vi "Delete Items.vi"(6 "indent":i32, 8 "error in (no error)":errorcluster, 9 "Copy? (F)":bool, 10 "Indices to remove":i32[](array[numeric]), 11 "BetterTreeHandle in":refnum<class "BetterTreeHandle.lvclass">) -> (0 "error out":errorcluster, 2 "Items removed":refnum<class "BetterItem.lvclass">[](array[class]), 3 "BetterTreeHandle out":refnum<class "BetterTreeHandle.lvclass">)   [LabVIEW 2020, in "BetterDragAndDrop.lvlib" / "BetterTreeHandle.lvclass"]
uses:
  BetterTreeHandle.lvclass
  C:/Code/GITHUB/BetterDragAndDrop/Source/Classes/BetterHandle/BetterHandle.lvclass
  BetterTreeItem/BetterItem.lvclass
  BetterHandle/BetterHandle.lvclass/BetterHandle.ctl
  BetterTreeHandle.lvclass/BetterTreeHandle.ctl
  1834b926-fef1-4190-b767-3c7c2e6ba27f.vi
  b5257fc7-a8b2-4340-9406-8318aee56996.vi
  1834b926-fef1-4190-b767-3c7c2e6ba27f.vi/bb9b305c-0eb3-4e25-bff2-b466a4ea47c4.vi
  b5257fc7-a8b2-4340-9406-8318aee56996.vi/bb9b305c-0eb3-4e25-bff2-b466a4ea47c4.vi
  BetterTreeItem/SubVIs/ReAnchor Steps POLY.vi
  BetterTreeItem/SubVIs/Re-Anchor steps TreeItemObjs.vi
  BetterTreeItem/SubVIs/Re-Anchor steps TreeItem.vi
  BetterHandle/BetterHandle.lvclass
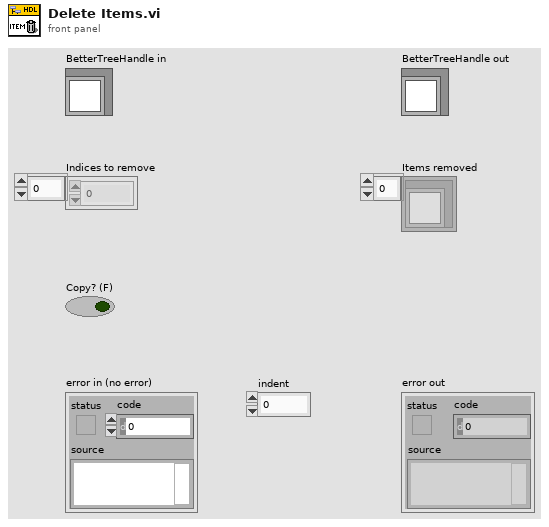
[diagram p1: front panel]
types:
  T1 = typedef "BetterDragAndDrop.lvlib/BetterTreeHandle.lvclass/TreeItem.ctl" = cluster{"Left Cell String":string, "Child Text":string[], "Child Tag":string, "Item Indent":i32, "Child Only?":bool, "Glyph Index":i32, "Font Color":u32}
  T2 = typedef "BetterDragAndDrop.lvlib/BetterTreeHandle.lvclass/Tree Move Indices.ctl" = cluster{"Parent Index":i32, "Children indices":i32[]}
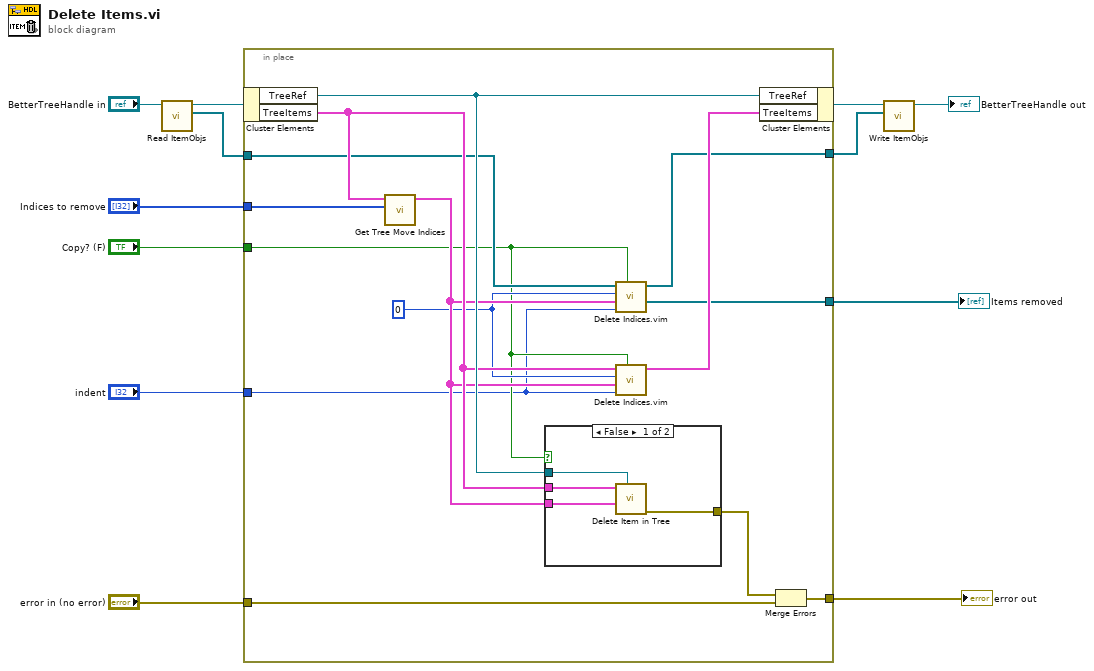
[diagram p0: block diagram]
diagram:
  n1 = call "Read ItemObjs.vi"("BetterHandle in"="BetterTreeHandle in") -> ("ItemObjs"=w8:refnum<class "BetterItem.lvclass">[], "BetterHandle out"=w11:refnum<class "BetterTreeHandle.lvclass">)  [unwired: 9 in]
  n2 = in-place {
    in-place-border: "error in (no error)" -> [w25]
    in-place-border: [w24] -> w5
    in-place-border: "Indices to remove" -> [w26]
    in-place-border: w8 -> [w18]
    in-place-border: [w17] -> w7
    in-place-border: [w15] -> w3
    in-place-border: "Copy? (F)" -> [w14]
    in-place-border: "indent" -> [w13]
    w16 = 0 ("indent")
    n3 = in-place-cluster #1(w11) -> ("TreeRef"=w23:refnum<vi>, "TreeItems"=w21:T1[])
    n4 = call "Get Tree Move Indices.vi"("Selected Indices"=w26, "TreeItems"=w21) -> ("Tree Move Indices"=w20:T2[])  [unwired: 9 in]
    n5 = case shown="False" w14 {
      tunnel: w23 -> [w30 _]
      tunnel: [w29 _] -> w22
      tunnel: w21 -> [w28 _]
      tunnel: w20 -> [w27 _]
      frame False {
        n6 = call "Delete Item in Tree.vi"("Tree ref"=w30, "Tree Move Indices"=w27, "TreeItems (current)"=w28) -> ("error out"=w29:errorcluster)  [unwired: 8 in]
      }
      frame True {
      }
    }
    n7 = call "Delete Indices.vim"("Copy?"=w14, "indent"=w13, "Tree Move Indices"=w20, "Insertion index"=w16, "TreeItems"=w18) -> ("elements to be inserted"=w15:refnum<class "BetterItem.lvclass">[], "TreeItems"=w17:refnum<class "BetterItem.lvclass">[])  [unwired: 4 in, 1 out]
    n8 = call "Delete Indices.vim"("Copy?"=w14, "indent"=w13, "Tree Move Indices"=w20, "Insertion index"=w16, "TreeItems"=w21) -> ("TreeItems"=w19:T1[])  [unwired: 4 in, 2 out]
    n9 = in-place-cluster #1("TreeRef"=w23, "TreeItems"=w19) -> (w9:refnum<class "BetterTreeHandle.lvclass">)
    n10 = Merge Errors(w22, w25) -> (w24:errorcluster)
  }
  "error out" <- w5
  "Items removed" <- w3
  n11 = call "Write ItemObjs.vi"("ItemObjs"=w7, "BetterHandle in"=w9) -> ("BetterHandle out"=→"BetterTreeHandle out":refnum<class "BetterTreeHandle.lvclass">)  [unwired: 9 in]
